vi "Send.vi"(5 "Record Topic Name?":bool, 7 "Message Priority":T1, 8 "error in (no error)":errorcluster, 9 "Timeout":i32, 10 "Message":refnum<class "Message Interface.lvclass">, 11 "Message Transport Event in":refnum<class "Message Transport Event.lvclass">) -> (0 "error out":errorcluster, 2 "Timed Out?":bool, 3 "Message Transport Event out":refnum<class "Message Transport Event.lvclass">)   [LabVIEW 2016, in "Stream Mediator.lvlib" / "Message Transport Event.lvclass"]
doc: "--\nCopyright © 2017 Composed SystemsI All rights reserved.\n\nAuthor: Jon McBee <jon.mcbee@composed.io>\n\nThis library is provided \"AS IS\" ,WITHOUT WARRANTIES OR\nCONDITIONS OF ANY KIND, either express or implied.\n\nComposed Systems -- composed.io\n\nStream 0.0.1.1\nJon McBee - Composed Systems\nCopyright (c) 2017, Composed Systems"
uses:
  <userlib>/Composed Systems/Stream/Mediator/Classes/Message Transport Event/Message Transport Event.lvclass
  C:/Program Files (x86)/National Instruments/LabVIEW 2016/user.lib/Composed Systems/Stream/Mediator/Classes/Message Transport Interface/Message Transport Interface.lvclass
  <userlib>/Composed Systems/Stream/Mediator/Classes/Message Interface/Message Interface.lvclass
  <userlib>/Composed Systems/Stream/Mediator/Classes/Message Transport Interface/Message Priority.ctl
  <userlib>/Composed Systems/Stream/Mediator/Classes/Message Interface/Message Interface.lvclass/Message Interface.ctl
  <userlib>/Composed Systems/Stream/Mediator/Classes/Message Transport Event/Message Transport Event.lvclass/Message Transport Event.ctl
  <vilib>/event_ctls.llb/usereventprio.ctl
  <userlib>/Composed Systems/Stream/Mediator/Classes/Message Transport Interface/Message Transport Interface.lvclass
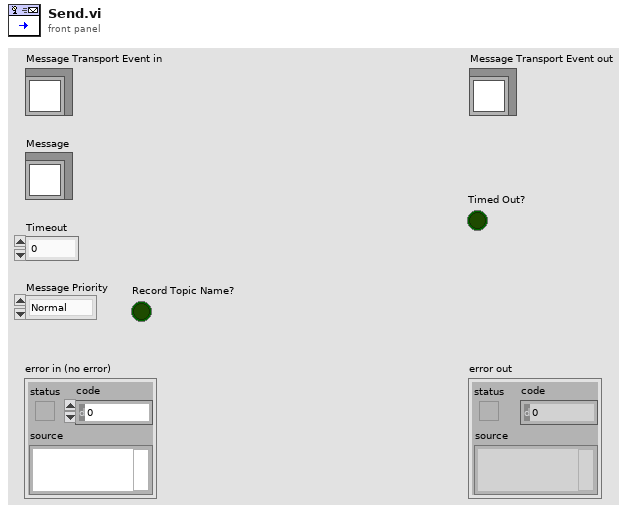
[diagram p1: front panel]
types:
  T1 = typedef "Stream Mediator.lvlib/Message Transport Interface.lvclass/Message Priority.ctl" = enum16{"Normal", "High"}
  T2 = typedef "usereventprio.ctl" = enum32{"high priority", "normal priority"}
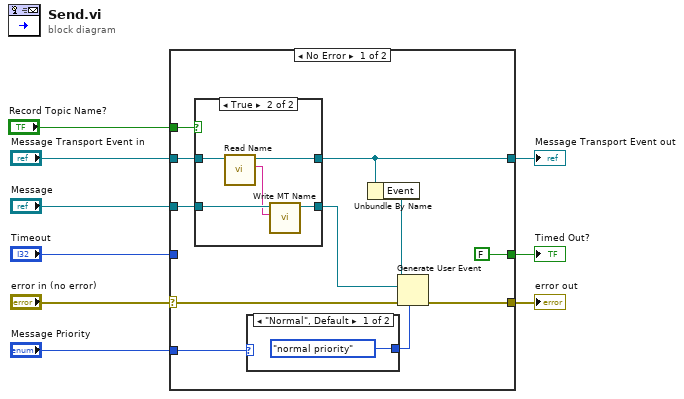
[diagram p0: block diagram]
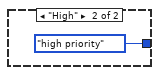
[diagram p3: hidden frame]
diagram:
  n1 = case shown="No Error" "error in (no error)" {
    selector: "error in (no error)" -> [w20 w30]
    tunnel: [w19 w30] -> w8
    tunnel: "Message" -> [w14 _]
    tunnel: [w11 w31] -> w6
    tunnel: "Message Transport Event in" -> [w12 w31]
    tunnel: "Timeout" -> [_ _]
    tunnel: [FALSE _] -> w3
    tunnel: "Message Priority" -> [w16 _]
    tunnel: "Record Topic Name?" -> [w10 _]
    frame No Error {
      n2 = case shown="True" w10 {
        tunnel: w14 -> [w21 w27]
        tunnel: [w21 w26] -> w13
        tunnel: w12 -> [w22 w25]
        tunnel: [w22 w24] -> w11
        frame False {
        }
        frame True {
          n3 = call <userlib>:"Read Name.vi"("Message Transport Interface in"=w25) -> ("Name"=w23:string, "Message Transport Interface out"=w24:refnum<class "Message Transport Event.lvclass">)  [unwired: 8 in, 1 out]
          n4 = call <userlib>:"Write MT Name.vi"("MT Name"=w23, "Message Interface in"=w27) -> ("Message Interface out"=w26:refnum<class "Message Interface.lvclass">)  [unwired: 9 in]
        }
      }
      n5 = case shown="\"Normal\", Default" w16 {
        tunnel: [usereventprio."normal priority" ("priority (normal)") usereventprio."high priority" ("priority (normal)")] -> w15
        frame "Normal", Default {
        }
        frame "High" {
        }
      }
      n6 = Unbundle By Name(w11) -> ("Event"=w18:refnum<user-event>)
      n7 = Generate User Event(priority (normal)=w15, user event=w18, event data cluster=w13, error in=w20) -> (error out=w19:errorcluster)  [unwired: 1 out]
    }
    frame Error {
    }
  }
  "error out" <- w8
  "Message Transport Event out" <- w6
  "Timed Out?" <- w3
